vi "DOEnableSet.vi"(0 "object in":refnum<class "AD2_DO_SDK.lvclass">, 2 "DOSingleCh":T1 {"IdleState" items=["PushPull", "OpenDrain", "OpenSource", "TriState"]; "DigitalOutOutput" items=["Pulse", "Custom", "Random"]; "Type" items=["Pulse", "Custom", "Random"]}, 5 "error in (no error)":errorcluster) -> (14 "object out":refnum<class "AD2_DO_SDK.lvclass">, 16 "DOSingleCh Out":T1 {"IdleState" items=["PushPull", "OpenDrain", "OpenSource", "TriState"]; "DigitalOutOutput" items=["Pulse", "Custom", "Random"]; "Type" items=["Pulse", "Custom", "Random"]}, 19 "error out":errorcluster)   [LabVIEW 2021, in "AD2_DO_SDK.lvclass"]
uses:
  AD2_DO_SDK.lvclass
  AD2_DO_SDK.lvclass/AD2_DO_SDK.ctl
  Olasdwf/Olasdwf.lvlib
  DOSingleCh.ctl
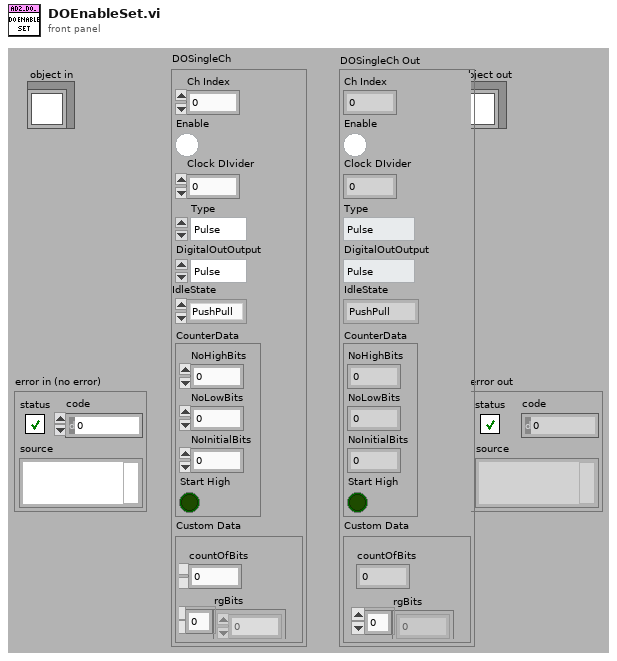
[diagram p1: front panel]
types:
  T1 = typedef "AD2_DO_SDK.lvclass/DOSingleCh.ctl" = cluster{"Ch Index":i32, "Enable":bool, "Clock DIvider":u32, "Type":i32, "DigitalOutOutput":u16, "IdleState":u16, "CounterData":cluster{"NoHighBits":u32, "NoLowBits":u32, "NoInitialBits":u32, "Start High":bool}, "Custom Data":cluster{"countOfBits":u32, "rgBits":u8[]}}
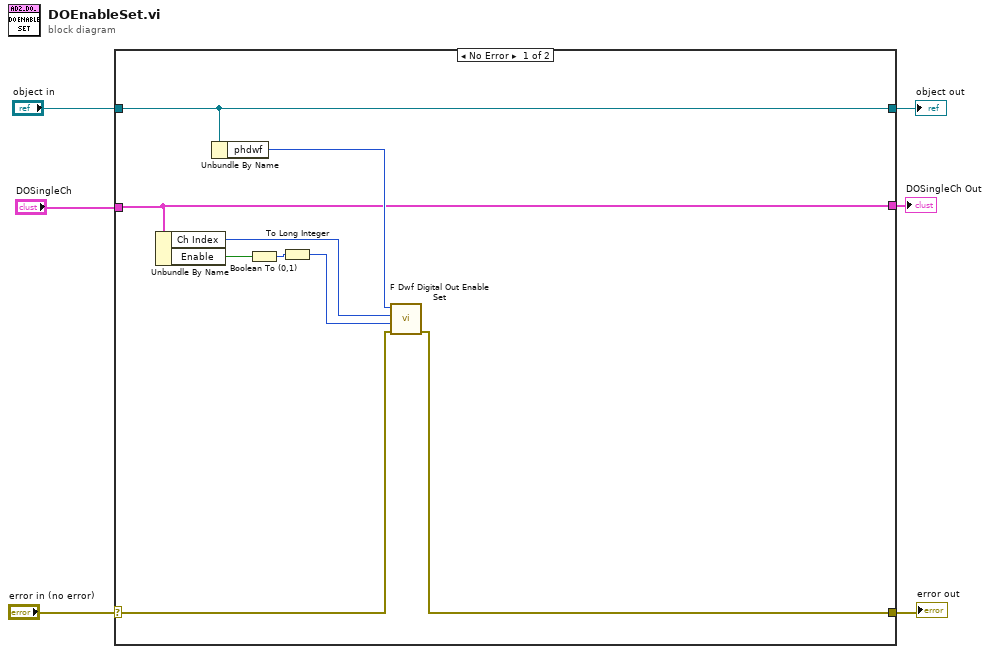
[diagram p0: block diagram]
diagram:
  n1 = case shown="No Error" "error in (no error)" {
    selector: "error in (no error)" -> [w13 w18]
    tunnel: [w12 w18] -> w5
    tunnel: [w15 w17] -> w3
    tunnel: "object in" -> [w15 w17]
    tunnel: "DOSingleCh" -> [w7 w16]
    tunnel: [w7 w16] -> w1
    frame No Error {
      n2 = Unbundle By Name(w7) -> ("Ch Index"=w11:i32, "Enable"=w8:bool)
      n3 = Unbundle By Name(w15) -> ("phdwf"=w14:i32)
      n4 = Boolean To (0,1)(Boolean=w8) -> (0, 1=w9:i16)
      n5 = To Long Integer(number=w9) -> (32bit integer=w10:i32)
      n6 = call "F Dwf Digital Out Enable Set.vi"("error in (no error)"=w13, "fEnable"=w10, "idxChannel"=w11, "hdwf"=w14) -> ("error out"=w12:errorcluster)  [unwired: 6 in, 1 out]
    }
    frame Error {
    }
  }
  "error out" <- w5
  "object out" <- w3
  "DOSingleCh Out" <- w1
